vi "Encoder_Noise.vi"(8 "dt_delta":dbl=0.001, 9 "dt(s)":dbl, 10 "True Position(rotations)":dbl, 11 "Position Offset Scalar":dbl=1.01) -> (1 "Measured Velocity(rotations/sec)":dbl, 2 "Measured Position(rotations)":dbl)   [LabVIEW 2019]
uses:
  <vilib>/numeric/Random Number (Range) DBL.vi
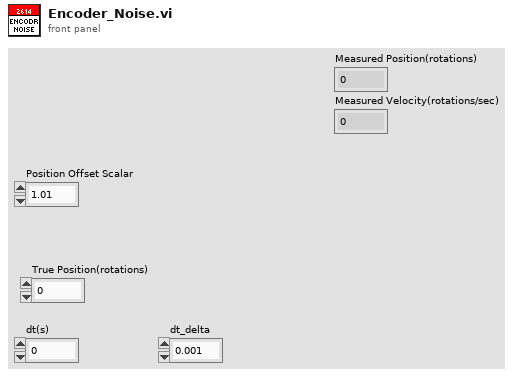
[diagram p1: front panel]
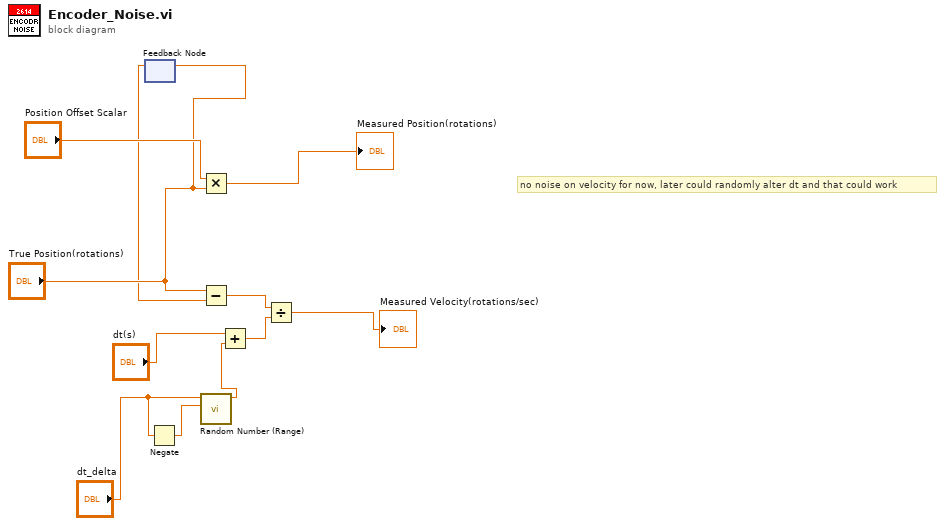
[diagram p0: block diagram]
diagram:
  # "no noise on velocity for now, later could randomly alter dt and that could work"
  n1 = feedback-in #1("True Position(rotations)") -> ()
  n2 = feedback #1() -> (w8:dbl)  [unwired: 1 in]
  n3 = Negate(x="dt_delta") -> (-x=w5:dbl)
  n4 = Multiply(x="Position Offset Scalar", y="True Position(rotations)") -> (x*y=→"Measured Position(rotations)":dbl)
  n5 = Subtract(x="True Position(rotations)", y=w8) -> (x-y=w7:dbl)
  n6 = call-poly <vilib>:"Random Number (Range).vi"("lower bound (0)"=w5, "upper bound (100)"="dt_delta") -> ("number"=w3:dbl)  [unwired: 9 in]
  n7 = Add(x="dt(s)", y=w3) -> (x+y=w6:dbl)
  n8 = Divide(x=w7, y=w6) -> (x/y=→"Measured Velocity(rotations/sec)":dbl)
